vi "RSZVB Configure Harmonic Measurement.vi"(4 "Relative Harmonic Measurement (F: Off)":bool, 5 "Harmonic Order (2)":i32=2, 6 "Harmonic Measured at (1)":i32=1, 7 "Source (1)":i32=1, 8 "error in (no error)":errorcluster {"code" format="%.0x"}, 9 "Harmonic Measurement (0: Off)":i32(ring)=1 items=["On"=1, "Off"=0], 10 "Channel (1)":i32=1, 11 "VISA session":refnum<visa-resource-name>) -> (0 "error out":errorcluster {"code" format="%.0x"}, 3 "dup VISA session":refnum<visa-resource-name>)   [LabVIEW 2011]
doc: "This VI configures the harmonic measurement on selected channel.\n\nRemote-control command(s):\n[SENSe<Ch>:]FREQuency:CONVersion FUNDamental | HARMonic\n[SENSe<Ch>:]FREQuency:CONVersion:HARMonic:ORDer\n[SENSe<Ch>:]FREQuency:CONVersion:HARMonic:SPORt\n[SENSe<Ch>:]FREQuency:CONVersion:HARMonic:RPORt\n[SENSe<Ch>:]FREQuency:CONVersion:HARMonic:RELative ON | OFF"
panel:
  # "On\nOff"
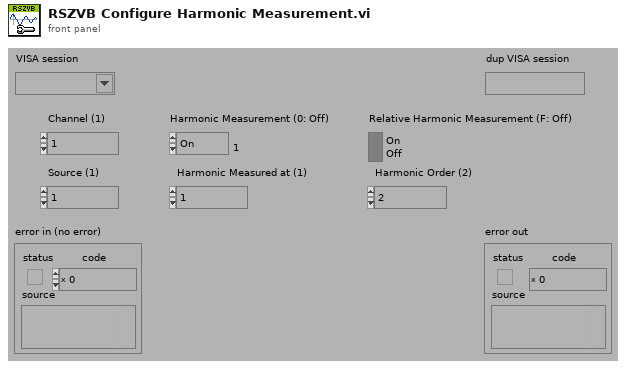
[diagram p1: front panel]
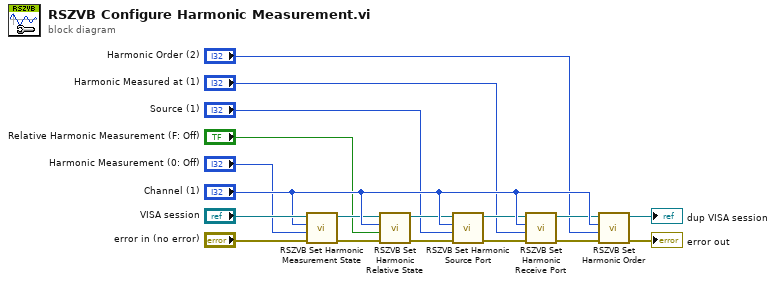
[diagram p0: block diagram]
diagram:
  n1 = call "RSZVB Set Harmonic Measurement State.vi"("error in (no error)"="error in (no error)", "Harmonic Measurement (0: Off)"="Harmonic Measurement (0: Off)", "Channel (1)"="Channel (1)", "VISA session"="VISA session") -> ("error out"=w18:errorcluster, "dup VISA session"=w6:refnum<visa-resource-name>)  [unwired: 6 in]
  n2 = call "RSZVB Set Harmonic Relative State.vi"("error in (no error)"=w18, "Relative Harmonic Measurement (F: Off)"="Relative Harmonic Measurement (F: Off)", "Channel (1)"="Channel (1)", "VISA session"=w6) -> ("error out"=w17:errorcluster, "dup VISA session"=w7:refnum<visa-resource-name>)  [unwired: 6 in]
  n3 = call "RSZVB Set Harmonic Source Port.vi"("error in (no error)"=w17, "Port (1)"="Source (1)", "Channel (1)"="Channel (1)", "VISA session"=w7) -> ("error out"=w16:errorcluster, "dup VISA session"=w8:refnum<visa-resource-name>)  [unwired: 6 in]
  n4 = call "RSZVB Set Harmonic Receive Port.vi"("error in (no error)"=w16, "Port (1)"="Harmonic Measured at (1)", "Channel (1)"="Channel (1)", "VISA session"=w8) -> ("error out"=w15:errorcluster, "dup VISA session"=w9:refnum<visa-resource-name>)  [unwired: 6 in]
  n5 = call "RSZVB Set Harmonic Order.vi"("error in (no error)"=w15, "Harmonic Order (2)"="Harmonic Order (2)", "Channel (1)"="Channel (1)", "VISA session"=w9) -> ("error out"=→"error out":errorcluster, "dup VISA session"=→"dup VISA session":refnum<visa-resource-name>)  [unwired: 6 in]
